vi "Pachube PUT EEML Format LaunchPad.vi"(10 "Pachube datastream ID":string="0", 11 "Value":string="25.0") -> (1 "Data":string)   [LabVIEW 2010]
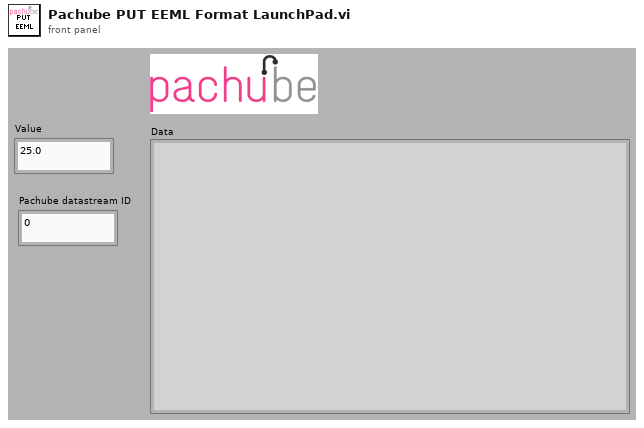
[diagram p1: front panel]
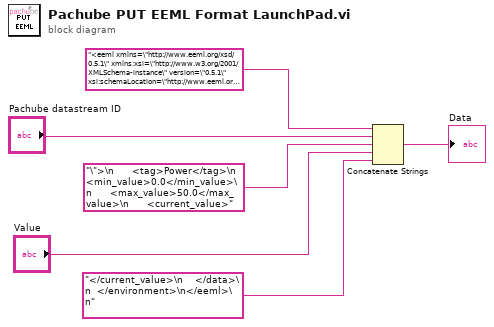
[diagram p0: block diagram]
diagram:
  n1 = Concatenate Strings("<eeml xmlns=\"http://www.eeml.org/xsd/0.5.1\" xmlns:xsi=\"http://www.w3.org/2001/XMLSchema-instance\" version=\"0.5.1\" xsi:schemaLocation=\"http://www.eeml.org/xsd/0.5.1 http://www.eeml.org/xsd/0.5.1/0.5.1.xsd\">\n  <environment>\n    <data id=\"", "Pachube datastream ID", "\">\n      <tag>Power</tag>\n      <min_value>0.0</min_value>\n      <max_value>50.0</max_value>\n      <current_value>", "Value", "</current_value>\n    </data>\n  </environment>\n</eeml>\n") -> (→"Data":string)
